vi "json_string.vi"(5 "text":string, 7 "ch":string, 9 "at":i32, 11 "error in (no error)":errorcluster) -> (4 "string":string, 6 "text dup":string, 8 "ch out":string, 10 "at":i32, 15 "error out":errorcluster)   [LabVIEW 2011]
doc: "Parse out a string typed JSON element."
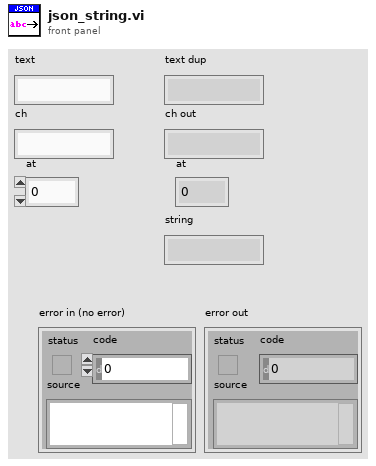
[diagram p1: front panel]
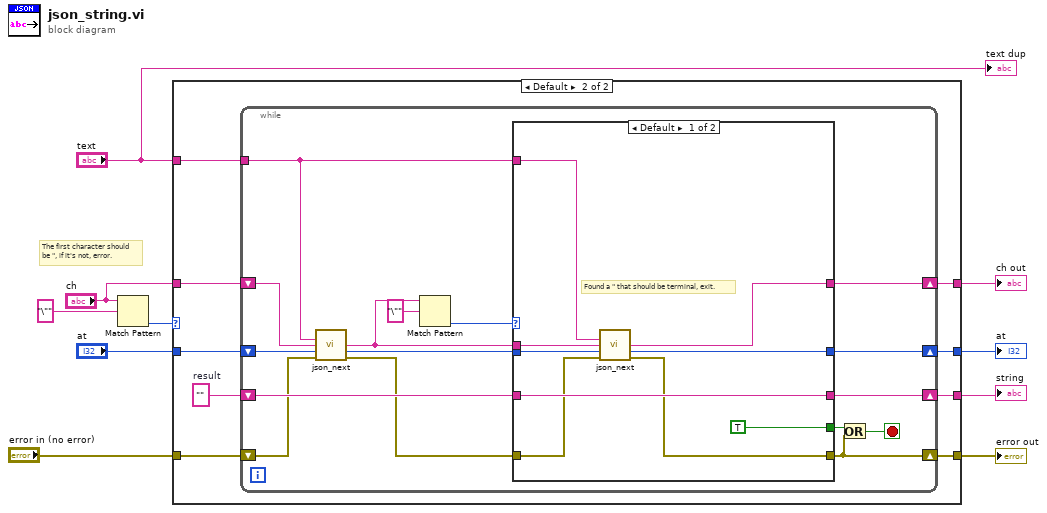
[diagram p0: block diagram]
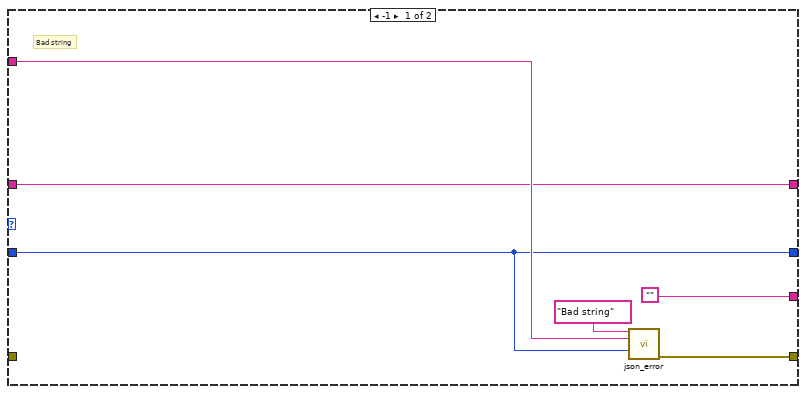
[diagram p2: hidden frame]
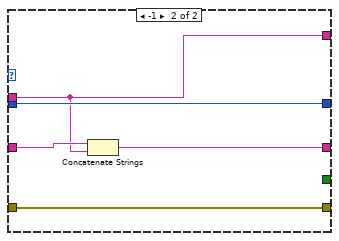
[diagram p3: hidden frame]
diagram:
  # "The first character should\nbe \", if it's not, error."
  n1 = Match Pattern(string="ch", regular expression="\"") -> (offset past match=w10:i32)  [unwired: 1 in, 3 out]
  n2 = case shown="Default" w10 {
    tunnel: "error in (no error)" -> [_ w21]
    tunnel: [w13 w22] -> w7
    tunnel: "text" -> [w16 w25]
    tunnel: "at" -> [w14 w24]
    tunnel: [w14 w23] -> w4
    tunnel: ["" w19] -> w3
    tunnel: [w12 w18] -> w2
    tunnel: "ch" -> [w12 w17]
    frame -1 {
      # "Bad string"
      n3 = call "json_error.vi"("m"="Bad string" ("source"), "text"=w16, "at"=w14) -> ("error out"=w13:errorcluster)  [unwired: 12 in]
    }
    frame Default {
      w20 = ""  # result
      n4 = while {
        tunnel: w25 -> [w36]
        shift-right: [w39] -> w23
        shift-left: w24 -> [w41]
        shift-right: [w28] -> w22
        shift-left: w21 -> [w31]
        shift-right: [w34] -> w19
        shift-left: w20 -> [w35]
        shift-right: [w32] -> w18
        shift-left: w17 -> [w29]
        stop <- w27 stop-if-true
        n5 = call "json_next.vi"("text"=w36, "ch"=w29, "at"=w41, "error in (no error)"=w31) -> ("ch out"=w33:string, "at out"=w38:i32, "error out"=w30:errorcluster)  [unwired: 8 in, 1 out]
        n6 = Match Pattern(string=w33, regular expression="\"") -> (offset past match=w37:i32)  [unwired: 1 in, 3 out]
        n7 = case shown="Default" w37 {
          tunnel: [w43 w55] -> w28
          tunnel: [w49 w54] -> w39
          tunnel: w38 -> [w50 w54]
          tunnel: w30 -> [w44 w55]
          tunnel: w36 -> [w48 _]
          tunnel: w35 -> [w47 w53]
          tunnel: [w47 w52] -> w34
          tunnel: w33 -> [w42 w51]
          tunnel: [TRUE _] -> w26
          tunnel: [w45 w51] -> w32
          frame Default {
            # "Found a \" that should be terminal, exit."
            n8 = call "json_next.vi"("text"=w48, "ch"=w42, "at"=w50, "error in (no error)"=w44) -> ("ch out"=w45:string, "at out"=w49:i32, "error out"=w43:errorcluster)  [unwired: 8 in, 1 out]
          }
          frame -1 {
            n9 = Concatenate Strings(w53, w51) -> (w52:string)
          }
        }
        n10 = Or(x=w26, y=w28) -> (x .or. y?=w27:bool)
      }
    }
  }
  "ch out" <- w2
  "at" <- w4
  "string" <- w3
  "error out" <- w7
  "text dup" <- "text"
